vi "Default Instrument Setup.vi"(8 "error in (no error)":errorcluster, 11 "VISA resource name":refnum<visa-resource-name>) -> (0 "error out":errorcluster, 3 "VISA resource name out":refnum<visa-resource-name>)   [LabVIEW 2019, in "Stanford Research SIM900 Series.lvlib"]
doc: "Sends a default command string to the instrument whenever a new VISA session is opened, or the instrument is reset. Use this VI as a subVI for the <b>Initialize</b> and <b>Reset</b> VIs. Altering this VI could cause these two VIs to operate incorrectly."
uses:
  Stanford Research SIM900 Series.lvlib
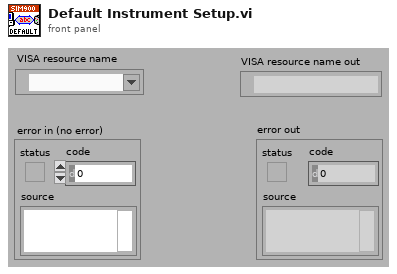
[diagram p1: front panel]
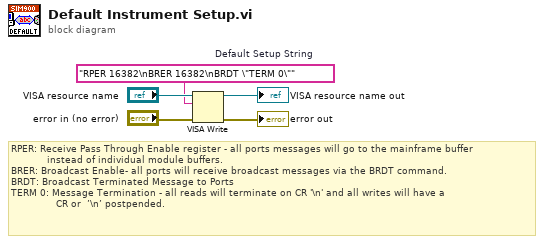
[diagram p0: block diagram]
diagram:
  w1 = "RPER 16382\nBRER 16382\nBRDT \"TERM 0\""  # Default Setup String
  # "RPER: Receive Pass Through Enable register - all ports messages will go to the mainframe buffer \n            instead of individual module buffers.\nBRER: Broadcast Enable- all ports will receive broadcast messages via the BRDT command.\nBRDT: Broadcast Terminated Message to Ports\nTERM 0: Message Termination - all reads will terminate on CR '\\n' and all writes will have a\n               CR or  ’\\n’ postpended."
  n1 = VISA Write(VISA resource name="VISA resource name", write buffer=w1, error in (no error)="error in (no error)") -> (VISA resource name out=→"VISA resource name out":refnum<visa-resource-name>, error out=→"error out":errorcluster)  [unwired: 1 out]
